vi "GetPathToPmuImpairPlugin.vi"(8 "ErrorArray In":errorcluster[](array[cluster]), 11 "Bus.lvclass In":refnum<class "Bus.lvclass">) -> (0 "ErrorArray Out":errorcluster[](array[cluster]), 2 "PmuImpairPluginINIFilePath":path, 3 "Bus.lvclass Out":refnum<class "Bus.lvclass">)   [LabVIEW 2014]
uses:
  <userlib>/NIST/NISTErrorLib/NISTErrorLib.lvlib
  <vilib>/Utility/error.llb/Error Cluster From Error Code.vi
  <vilib>/ErrorRing/Error Ring.xnode
  Bus.lvclass
  PmuImpairment/PmuImpairModule/PmuImpairModule.lvlib
  PmuImpairment/PmuImpairModule/PublicAPI/Arguments/Requests/clLoadPlugin.ctl
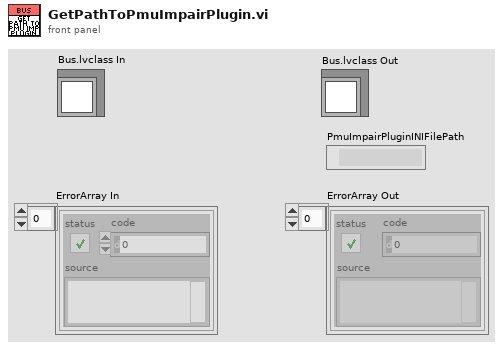
[diagram p1: front panel]
types:
  T1 = typedef "PmuImpairModule.lvlib/clBroadcastEvents.ctl" = cluster{"DidInit":refnum<user-event>, "StatusUpdate":refnum<user-event>, "ErrorReport":refnum<user-event>, "DidStop":refnum<user-event>, "ImpairConfig":refnum<user-event>, "ImpairParams":refnum<user-event>, "ImpairReports":refnum<user-event>, "PathToPlugin":refnum<user-event>, "BusNumber":refnum<user-event>}
  T2 = typedef "PmuImpairModule.lvlib/clLoadPlugin.ctl" = cluster{"PathToPlugin":path}
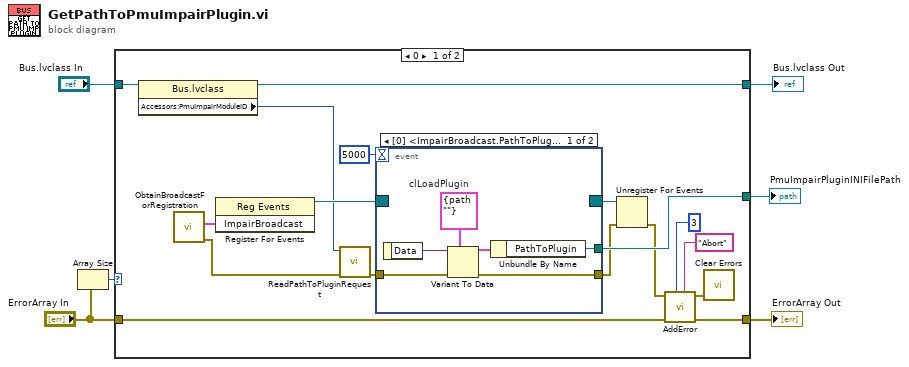
[diagram p0: block diagram]
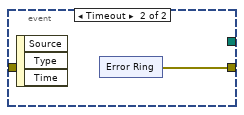
[diagram p2: hidden frame]
diagram:
  n1 = Array Size(array="ErrorArray In") -> (size(s)=w5:i32)
  n2 = case shown="0" w5 {
    tunnel: "ErrorArray In" -> [w23 w37]
    tunnel: [w22 w37] -> w6
    tunnel: "Bus.lvclass In" -> [w18 w36]
    tunnel: [w12 w36] -> w2
    tunnel: [w11 _] -> w1
    frame 0 {
      n3 = property class="Bus.lvclass"(reference=w18) -> (reference out=w12:refnum<class "Bus.lvclass">, "Accessors:PmuImpairModuleID"=w13:i32)  [unwired: 1 in, 1 out]
      n4 = call "ObtainBroadcastForRegistration.vi"() -> ("error out"=w15:errorcluster, "ImpairBroadcast"=w17:T1)  [unwired: 10 in]
      n5 = register-events(w17) -> (reference out=w16:refnum<event-registration>)  [unwired: 2 in, 1 out]
      n6 = call "ReadPathToPluginRequest.vi"("error in (no error)"=w15, "ModuleID"=w13) -> ("error out"=w14:errorcluster)  [unwired: 9 in]
      n7 = event shown="[0] <ImpairBroadcast.PathToPlugin>: User Event" {
        selector: w16 -> [_ _]
        dyn-events: [_ _] -> w9
        timeout: 5000 -> [_ _]
        tunnel: w14 -> [w28 _]
        tunnel: [w25 _] -> w11
        tunnel: [w24 w30] -> w7
        event User Event {
          w27 = T2 {"PathToPlugin"=path ""}  # clLoadPlugin
          n8 = event-data() -> ("Data"=w29:variant)  [unwired: 1 in]
          n9 = Variant To Data(error in=w28, type=w27, Variant=w29) -> (data=w26:T2, error out=w24:errorcluster)
          n10 = Unbundle By Name(w26) -> ("PathToPlugin"=w25:path)
        }
        event Timeout {
          n11 = event-data() -> ()  [unwired: 1 in, 3 out]
          n12 = xnode "Error Ring"() -> ("error out"=w30:errorcluster)
        }
      }
      n13 = Unregister For Events(event registration refnum=w9, error in=w7) -> (error out=w8:errorcluster)
      n14 = call <userlib>:"AddError.vi"("Severity"="Abort" ("String"), "Priority"=u8 3, "ErrorArray"=w23, "error in (no error)"=w8) -> ("ErrorArray"=w22:errorcluster[], "error out"=w21:errorcluster)  [unwired: 6 in]
      n15 = call <vilib>:"Clear Errors.vi"("error in (no error)"=w21) -> ()  [unwired: 5 in, 2 out]
    }
    frame 1, Default {
    }
  }
  "ErrorArray Out" <- w6
  "Bus.lvclass Out" <- w2
  "PmuImpairPluginINIFilePath" <- w1
